vi "Agilent 34401 Read Math Measurement.vi"() -> ()   [LabVIEW 2012]
doc: "This example shows how to configure a Math measurement and take multiple readings."
uses:
  <vilib>/Utility/error.llb/DialogType.ctl
  <instrlib>/Agilent 34401/Public/Data/Read (Multiple Points).vi
  <instrlib>/Agilent 34401/Public/Data/Read (Math).vi
  <instrlib>/Agilent 34401/Agilent 34401.lvlib
panel:
  out "Standard Deviation":dbl
  out "Peak-to-Peak":dbl
  out "Count":dbl
  out "Average":dbl
  out "Minimum":dbl
  out "Maximum":dbl
  in  "Reset After Read (False)":bool
  in  "Lower Limit (0.00)":dbl format="%.2f"
  in  "Upper Limit (0.00)":dbl format="%.2f"
  in  "dBm Resistance (600 Ohms)":i32(ring)=600 items=["50"=50, "75"=75, "93"=93, "110"=110, "124"=124, "125"=125, "135"=135, "150"=150, "250"=250, "300"=300, "500"=500, "600"=600, "800"=800, "900"=900, "1000"=1000, "1200"=1200, "8000"=8000]
  in  "dB Reference Point (0.00 dB)":dbl format="%.2f"
  out "Measurements":dbl[](array[numeric])
  in  "Null Offset (0.00)":dbl format="%_3f"
  in  "Operation (0:None)":T1(ring)
  in  "Function (0: DC Voltage)":u16(ring) items=["DC Voltage", "AC Voltage", "2 - Wire Resistance", "4 - Wire Resistance", "DC Current", "AC Current", "Frequency", "Period", "Continuity", "Diode Checking", "VDC:VDC Ratio", "Temperature", "Capacitance"]
  in  "Enable Auto Range (T: Enable)":bool=TRUE
  in  "Manual Resolution (5.5 Digits)":dbl(ring)=5.5 items=["4.5"=4.5, "5.5"=5.5, "6.5"=6.5]
  in  "Manual Range (1.00)":dbl=1.0 format="%_3f"
  in  "Serial Configuration":T2={"Baud Rate"=9600, "Parity"=2, "Data Bits"=7} {"Data Bits" items=["7"=7, "8"=8]; "Parity" items=["None", "Odd", "Even"]; "Baud Rate" items=["300"=300, "600"=600, "1200"=1200, "2400"=2400, "4800"=4800, "9600"=9600, "19200"=19200]}
  in  "VISA resource name":refnum<visa-resource-name>
  # "(c) 2005-2008 National Instruments.  ALL RIGHTS RESERVED."
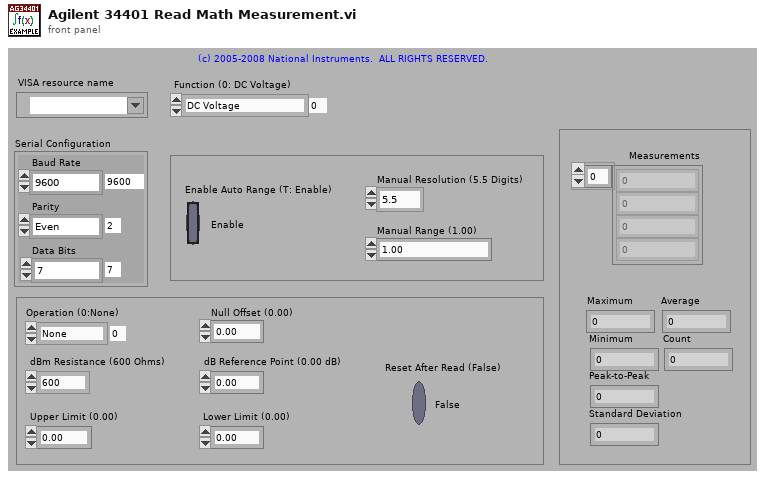
[diagram p1: front panel]
types:
  T1 = enum16{"None", "Min/Max", "Null", "dB", "dBm", "Limit"}
  T2 = cluster{"Baud Rate":u32, "Parity":u16, "Data Bits":u16}
  T3 = typedef "DialogType.ctl" = u16
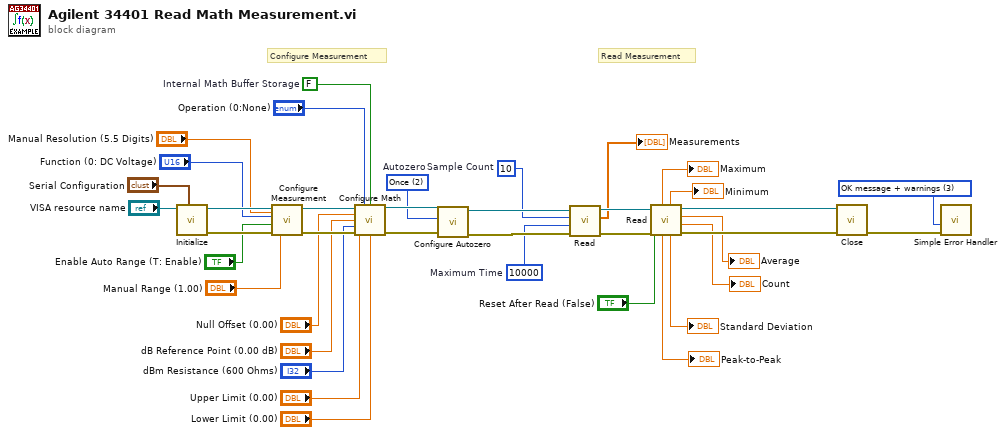
[diagram p0: block diagram]
diagram:
  w12 = u32 10000  # Maximum Time
  w14 = 10  # Sample Count
  w17 = FALSE  # Internal Math Buffer Storage
  w16 = u16 2 items=["On", "Off", "Once"]  # Autozero
  w27 = T3 3 items=["no dialog", "OK message", "continue or stop message", "OK message + warnings", "continue/stop + warnings"] ("type of dialog (OK msg:1)")
  # "Read Measurement"
  # "Configure Measurement"
  n1 = call <instrlib>:"Initialize.vi"("Serial Configuration"="Serial Configuration", "VISA resource name"="VISA resource name") -> ("error out"=w32:errorcluster, "VISA resource name out"=w33:refnum<visa-resource-name>)  [unwired: 8 in]
  n2 = call <instrlib>:"Configure Measurement.vi"("Manual Range (1.00)"="Manual Range (1.00)", "Manual Resolution (5.5 Digits)"="Manual Resolution (5.5 Digits)", "error in (no error)"=w32, "Enable Auto Range (T: Enable)"="Enable Auto Range (T: Enable)", "Function (0: DC Voltage)"="Function (0: DC Voltage)", "VISA resource name"=w33) -> ("error out"=w25:errorcluster, "VISA resource name out"=w26:refnum<visa-resource-name>)  [unwired: 4 in]
  n3 = call <instrlib>:"Configure Math.vi"("VISA resource name"=w26, "Operation (0:None)"="Operation (0:None)", "Internal Math Buffer Storage (T: Enabled)"=w17, "Null Offset (0.00)"="Null Offset (0.00)", "dB Reference Point (0.00 dB)"="dB Reference Point (0.00 dB)", "dBm Resistance (600 Ohms)"="dBm Resistance (600 Ohms)", "error in (no error)"=w25, "Upper Limit (0.00)"="Upper Limit (0.00)", "Lower Limit (0.00)"="Lower Limit (0.00)") -> ("VISA resource name out"=w24:refnum<visa-resource-name>, "error out"=w23:errorcluster)  [unwired: 5 in]
  n4 = call <instrlib>:"Configure Autozero.vi"("error in (no error)"=w23, "Autozero  (0: On)"=w16, "VISA resource name"=w24) -> ("error out"=w21:errorcluster, "VISA resource name out"=w22:refnum<visa-resource-name>)  [unwired: 7 in]
  n5 = call-poly <instrlib>:"Read.vi"("error in (no error)"=w21, "Maximum Time (10000 ms)"=w12, "Sample Count (1)"=w14, "VISA resource name"=w22) -> ("error out"=w19:errorcluster, "Measurements"=→"Measurements":dbl[], "VISA resource name out"=w20:refnum<visa-resource-name>)  [unwired: 5 in]
  n6 = call-poly <instrlib>:"Read.vi"("error in (no error)"=w19, "Reset After Read (False)"="Reset After Read (False)", "VISA resource name"=w20) -> ("error out"=w35:errorcluster, "Count"=→"Count":dbl, "Average"=→"Average":dbl, "VISA resource name out"=w34:refnum<visa-resource-name>, "Standard Deviation"=→"Standard Deviation":dbl, "Minimum"=→"Minimum":dbl, "Peak-to-Peak"=→"Peak-to-Peak":dbl, "Maximum"=→"Maximum":dbl)  [unwired: 1 in]
  n7 = call <instrlib>:"Close.vi"("error in (no error)"=w35, "VISA resource name"=w34) -> ("error out"=w38:errorcluster)  [unwired: 9 in]
  n8 = call <vilib>:"Simple Error Handler.vi"("type of dialog (OK msg:1)"=w27, "error in (no error)"=w38) -> ()  [unwired: 3 in, 5 out]
